vi "CMC_Debug_Exercise_(Main).vi"() -> ()   [LabVIEW 2013]
doc: "This exercise is used to demonstrate the use of different debugging tools."
panel:
  out "Final Result":dbl format="%.2f"
  out "Random Number":dbl format="%.2f"
  out "Multiply Result":dbl format="%.2f"
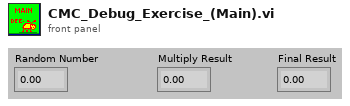
[diagram p1: front panel]
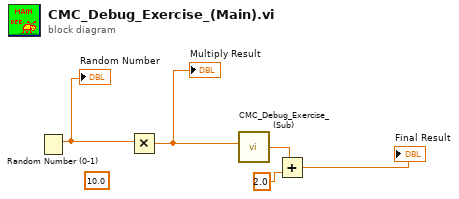
[diagram p0: block diagram]
diagram:
  (unwired) 10.0
  n1 = Random Number (0-1)() -> (number: 0 to 1=w4:dbl)
  "Random Number" <- w4
  n2 = Multiply(x=w4) -> (x*y=w5:dbl)  [unwired: 1 in]
  "Multiply Result" <- w5
  n3 = call "CMC_Debug_Exercise_(Sub).vi"("Number"=w5) -> ("Final Result"=w2:dbl)
  n4 = Add(x=w2, y=2.0) -> (x+y=→"Final Result":dbl)
